vi "Check Status.vi"(8 "error in (no error)":errorcluster, 11 "MicrowaveAmp in":refnum<class "MicrowaveAmp.lvclass">) -> (0 "error out":errorcluster, 1 "Status":string, 2 "Ready?":bool, 3 "MicrowaveAmp out":refnum<class "MicrowaveAmp.lvclass">)   [LabVIEW 2009, in "MicrowaveAmp.lvclass"]
doc: "(Dynamic) Check if the instrument is powered on and update its member fields with the instrument's current status. Optionally return a text status message."
uses:
  MicrowaveAmp.lvclass
  Utility Classes/Scannable/Scannable.lvclass
  MicrowaveAmp.lvclass/MicrowaveAmp.ctl
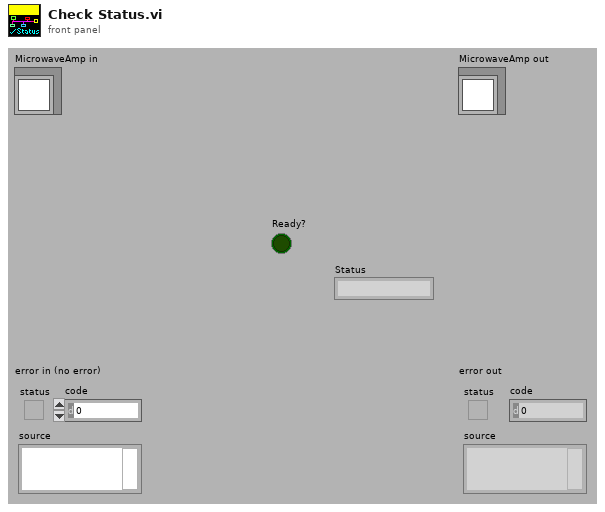
[diagram p1: front panel]
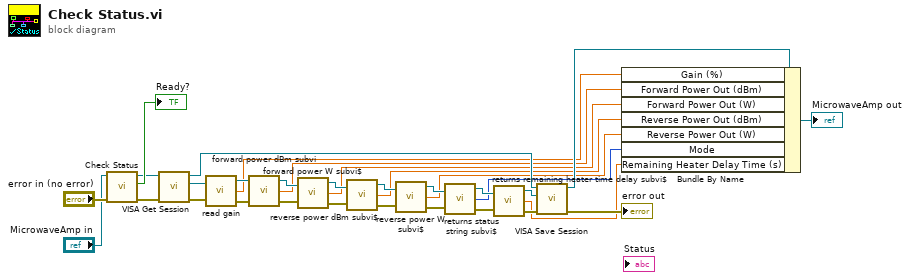
[diagram p0: block diagram]
diagram:
  n1 = call-parent "Check Status.vi"("error in (no error)"="error in (no error)", "Instrument in"="MicrowaveAmp in") -> ("error out"=w11:errorcluster, "Ready?"=→"Ready?":bool, "Instrument out"=w23:refnum<class "MicrowaveAmp.lvclass">)  [unwired: 6 in, 1 out]
  n2 = call-dynamic "VISA Get Session.vi"("error in (no error)"=w11, "Instrument.lvclass in"=w23) -> ("error out"=w12:errorcluster, "VISA Resource Name"=w22:refnum<visa-resource-name>, "Instrument.lvclass out"=w10:refnum<class "MicrowaveAmp.lvclass">)  [unwired: 7 out]
  n3 = call "read gain.vi"("VISA resource name"=w22, "error in (no error)"=w12) -> ("VISA resource name out"=w21:refnum<visa-resource-name>, "Gain (%)"=w7:dbl, "error out"=w29:errorcluster)
  n4 = call "forward power dBm subvi.vi"("error in (no error)"=w29, "VISA resource name"=w21) -> ("error out"=w28:errorcluster, "forward power (dBm)"=w6:dbl, "VISA resource name out"=w20:refnum<visa-resource-name>)  [unwired: 1 in]
  n5 = call "forward power W subvi$.vi"("VISA resource name"=w20, "error in (no error)"=w28) -> ("VISA resource name out"=w19:refnum<visa-resource-name>, "foward power (W)"=w5:dbl[unit], "error out"=w27:errorcluster)
  n6 = call "reverse power dBm subvi$.vi"("VISA resource name"=w19, "error in (no error)"=w27) -> ("VISA resource name out"=w18:refnum<visa-resource-name>, "reverse power (dBm)"=w4:dbl, "error out"=w26:errorcluster)
  n7 = call "reverse power W subvi$.vi"("VISA resource name"=w18, "error in (no error)"=w26) -> ("VISA resource name out"=w17:refnum<visa-resource-name>, "Reverse Power (W)"=w3:dbl[unit], "error out"=w25:errorcluster)
  n8 = call "returns status string subvi$.vi"("VISA resource name"=w17, "error in (no error)"=w25) -> ("VISA resource name out"=w16:refnum<visa-resource-name>, "Mode"=w2:u16, "error out"=w24:errorcluster)
  n9 = call "returns remaining heater time delay subvi$.vi"("VISA resource name"=w16, "error in (no error)"=w24) -> ("VISA resource name out"=w15:refnum<visa-resource-name>, "Heater delay time (s)"=w1:dbl[unit], "error out"=w14:errorcluster)
  n10 = call-dynamic "VISA Save Session.vi"("error in (no error)"=w14, "VISA Resource Name"=w15, "Instrument.lvclass in"=w10) -> ("error out"=→"error out":errorcluster, "Instrument.lvclass out"=w9:refnum<class "MicrowaveAmp.lvclass">)  [unwired: 7 out]
  n11 = Bundle By Name(cluster=w9, "Gain (%)"=w7, "Forward Power Out (dBm)"=w6, "Forward Power Out (W)"=w5, "Reverse Power Out (dBm)"=w4, "Reverse Power Out (W)"=w3, "Mode"=w2, "Remaining Heater Delay Time (s)"=w1) -> (→"MicrowaveAmp out":refnum<class "MicrowaveAmp.lvclass">)
